vi "Configure Error Checking.vi"(7 "Status Checking (On)":bool=TRUE, 8 "error in (no error)":errorcluster, 9 "Range Checking (On)":bool=TRUE, 10 "Option Checking (On)":bool=TRUE, 11 "VISA resource name":refnum<visa-resource-name>) -> (0 "error out":errorcluster, 3 "VISA resource name out":refnum<visa-resource-name>)   [LabVIEW 2020, in "Rohde&Schwarz CMWXP NR FR1 Measurement.lvlib"]
doc: "This VI combines into one the settings performed by the following VIs:\n<b>Instrument Status Checking.vi</b>, <b>Range Checking.vi</b>, <b>Option Checking.vi</b>\n\nThe default state for all three settings after initializing the session is <b>ON</b>."
uses:
  <instrlib>/Rohde&Schwarz CMWXP NR FR1 Measurement/Rohde&Schwarz CMWXP NR FR1 Measurement.lvlib
  <instrlib>/Rohde&Schwarz CMWXP NR FR1 Measurement/Private/rsidr_core.llb/type_Session_Parameter_boolean.ctl
  <instrlib>/Rohde&Schwarz CMWXP NR FR1 Measurement/Private/rsidr_core.llb/rsidr_core.lvlib
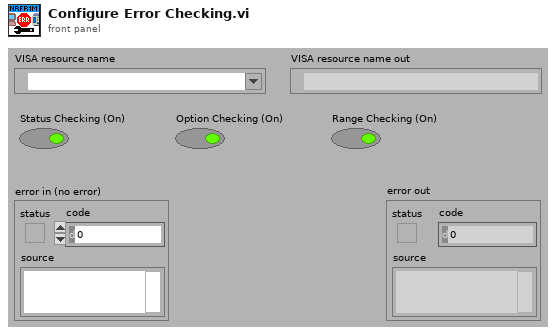
[diagram p1: front panel]
types:
  T1 = typedef "Rohde&Schwarz CMWXP NR FR1 Measurement.lvlib/rsidr_core.lvlib/type_Session_Parameter_boolean.ctl" = enum16{"Simulate", "Query Instr Status", "Check Range", "Check Options", "Add LF to Write", "Duplicate Session", "Fast Sweep", "Logging"}
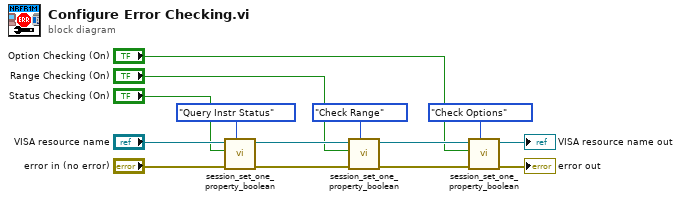
[diagram p0: block diagram]
diagram:
  n1 = call <instrlib>:"session_set_one_property_boolean.vi"("Session Parameter boolean"=type_Session_Parameter_boolean."Query Instr Status", "error in"="error in (no error)", "boolean value in"="Status Checking (On)", "VISA resource name"="VISA resource name") -> ("error out"=w12:errorcluster, "VISA resource name out"=w11:refnum<visa-resource-name>)  [unwired: 5 in, 1 out]
  n2 = call <instrlib>:"session_set_one_property_boolean.vi"("Session Parameter boolean"=type_Session_Parameter_boolean."Check Range", "error in"=w12, "boolean value in"="Range Checking (On)", "VISA resource name"=w11) -> ("error out"=w10:errorcluster, "VISA resource name out"=w9:refnum<visa-resource-name>)  [unwired: 5 in, 1 out]
  n3 = call <instrlib>:"session_set_one_property_boolean.vi"("Session Parameter boolean"=type_Session_Parameter_boolean."Check Options", "error in"=w10, "boolean value in"="Option Checking (On)", "VISA resource name"=w9) -> ("error out"=→"error out":errorcluster, "VISA resource name out"=→"VISA resource name out":refnum<visa-resource-name>)  [unwired: 5 in, 1 out]
